vi "SR400 ErrorHandler.vi"(2 "error in (no error)":errorcluster, 3 "Status Code":u8) -> (0 "error out":errorcluster, 1 "Erreur":bool)   [LabVIEW 2019]
doc: "Ce VI vérifie si une erreur a eu lieu et si c'est le cas, il affiche un message. Si l'erreur provient du contrôleur, celle-ci est ensuite effacée."
uses:
  <vilib>/Utility/error.llb/DialogType.ctl
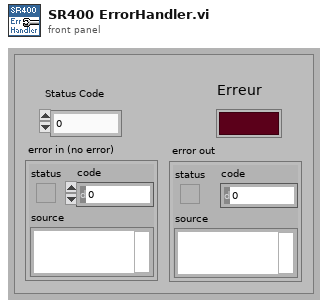
[diagram p1: front panel]
types:
  T1 = typedef "DialogType.ctl" = u16
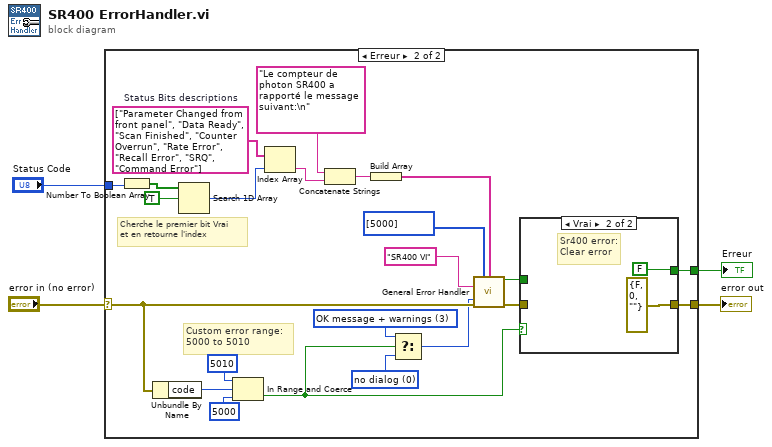
[diagram p0: block diagram]
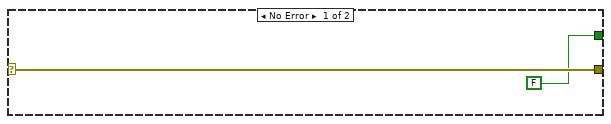
[diagram p2: hidden frame]
diagram:
  n1 = case shown="Erreur" "error in (no error)" {
    selector: "error in (no error)" -> [w6 w10]
    tunnel: [w6 w25] -> w4
    tunnel: [FALSE ("error?") w22] -> w3
    tunnel: "Status Code" -> [_ w20]
    frame No Error {
    }
    frame Error {
      w11 = T1 0 items=["no dialog", "OK message", "continue or stop message", "OK message + warnings", "continue/stop + warnings"] ("type of dialog (OK msg:1)")
      w12 = T1 3 items=["no dialog", "OK message", "continue or stop message", "OK message + warnings", "continue/stop + warnings"] ("type of dialog (OK msg:1)")
      w27 = string[] ["Parameter Changed from front panel", "Data Ready", "Scan Finished", "Counter Overrun", "Rate Error", "Recall Error", "SRQ", "Command Error"]  # Status Bits descriptions
      # "Cherche le premier bit Vrai\net en retourne l'index"
      # "Custom error range:\n5000 to 5010"
      n2 = Number To Boolean Array(number=w20) -> (Boolean array=w19:bool[])
      n3 = Unbundle By Name(w10) -> ("code"=w9:i32)
      n4 = Search 1D Array(1D array=w19, element=TRUE) -> (index of element=w17:i32)  [unwired: 1 in]
      n5 = In Range and Coerce(upper limit=5010, x=w9, lower limit=5000) -> (In Range?=w7:bool)  [unwired: 1 out]
      n6 = Index Array(array=w27, index=w17) -> (element=w15:string)
      n7 = Concatenate Strings("Le compteur de photon SR400 a rapporté le message suivant:\n" ("string"), w15) -> (w14:string)
      n8 = Build Array(w14) -> (w13:string[])
      n9 = Select(t=w12, s=w7, f=w11) -> (s? t:f=w8:T1)
      n10 = call <vilib>:"General Error Handler.vi"("[user-defined codes]"=i32[] [5000], "[user-defined descriptions]"=w13, "[error source] (\" \")"="SR400 VI" ("[error source] (\" \")"), "type of dialog (OK msg:1)"=w8, "error in (no error)"=w10) -> ("error?"=w21:bool, "error out"=w26:errorcluster)  [unwired: 6 in, 3 out]
      n11 = case shown="Vrai" w7 {
        tunnel: [w31 errorcluster {"status"=FALSE, "code"=0, "source"=""} ("error out")] -> w25
        tunnel: w26 -> [w31 _]
        tunnel: [w30 FALSE ("error?")] -> w22
        tunnel: w21 -> [w30 _]
        frame False {
          # "Not a Sr400 error:\nPass error out"
        }
        frame True {
          # "Sr400 error:\nClear error"
        }
      }
    }
  }
  "Erreur" <- w3
  "error out" <- w4
